vi "ATSpectrograph_salCommander_disable.vi"(8 "error in (no error)":errorcluster) -> (0 "error out":errorcluster, 3 "function return":i32)   [LabVIEW 2016, in "SALLV_ATSpectrograph.lvlib"]
doc: "int ATSpectrograph_shm_salCommander_disableLV();"
uses:
  SALLV_ATSpectrograph.lvlib
  SALLV_ATSpectrograph.so
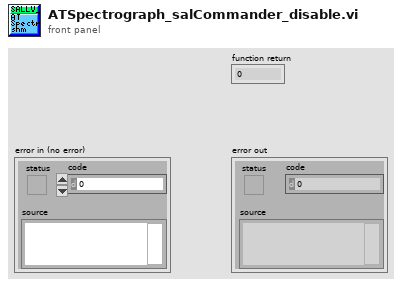
[diagram p1: front panel]
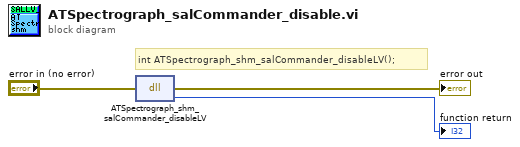
[diagram p0: block diagram]
diagram:
  # "int ATSpectrograph_shm_salCommander_disableLV();"
  n1 = dll-call lib="home/harini/tcs/ts_AtSpectrograph/ts_sallv_AtSpectrograph/SALLV_ATSpectrograph.*" fn="ATSpectrograph_shm_salCommander_disableLV"(error in="error in (no error)") -> (error out=→"error out":errorcluster, →"function return":i32)  [unwired: 2 in, 1 out]
